vi "Initialize Motor Communication Ref.vi"(8 "error in (no error)":errorcluster, 11 "motor name (unnamed)":string) -> (0 "error out":errorcluster, 3 "motor communication ref out":refnum<class "NI_Robotics_Motor Communication Ref.lvclass">)   [LabVIEW 2017, in "NI_Robotics_Motor Communication Ref.lvclass"]
uses:
  <vilib>/robotics/Actuation/Motor Communication Ref/NI_Robotics_Motor Communication Ref.lvclass
  c:/Program Files (x86)/National Instruments/LabVIEW 2017/vi.lib/robotics/Actuation/Motor Communication/NI_Robotics_Motor Communication.lvclass
  <vilib>/robotics/Actuation/Motor Communication Ref/NI_Robotics_Motor Communication Ref.lvclass/NI_Robotics_Motor Communication Ref.ctl
  <vilib>/robotics/Actuation/Motor Communication/NI_Robotics_Motor Communication.lvclass/NI_Robotics_Motor Communication.ctl
  <vilib>/robotics/Actuation/Motor Communication Ref/FG Motor Comm Ref Sessions Action.ctl
  <vilib>/robotics/Actuation/Motor Communication Ref/Check if Refs are Valid.vi
  <vilib>/robotics/Actuation/Motor Communication/NI_Robotics_Motor Communication.lvclass
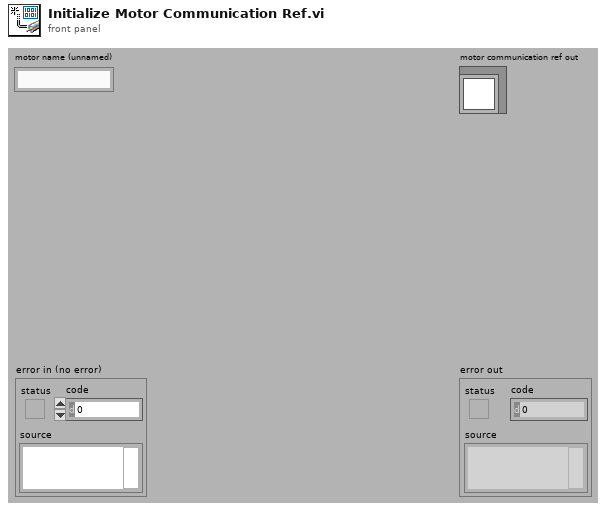
[diagram p1: front panel]
types:
  T1 = typedef "NI_Robotics_Motor Communication Ref.lvclass/FG Motor Comm Ref Sessions Action.ctl" = enum16{"Get", "Add", "Delete"}
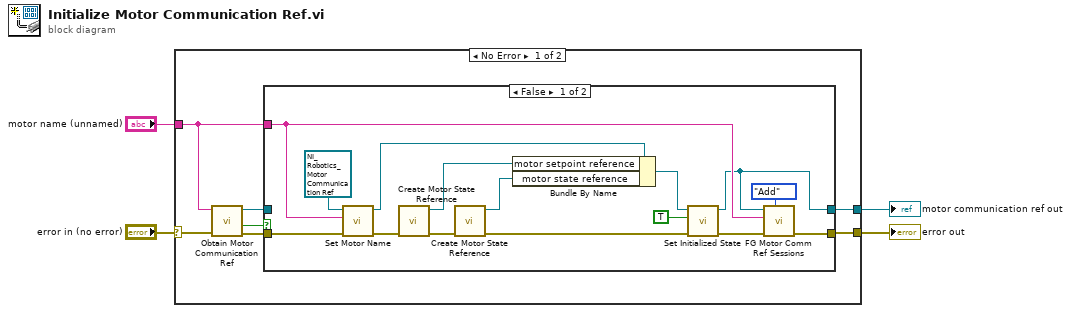
[diagram p0: block diagram]
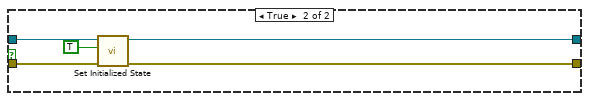
[diagram p2: hidden frame]
diagram:
  n1 = case shown="No Error" "error in (no error)" {
    selector: "error in (no error)" -> [w7 w32]
    tunnel: [w8 w32] -> w3
    tunnel: "motor name (unnamed)" -> [w6 _]
    tunnel: [w5 _] -> w1
    frame No Error {
      n2 = call <vilib>:"Obtain Motor Communication Ref.vi"("error in (no error)"=w7, "motor name"=w6) -> ("error out"=w10:errorcluster, "valid?"=w11:bool, "motor communication ref out"=w9:refnum<class "NI_Robotics_Motor Communication Ref.lvclass">)  [unwired: 7 in]
      n3 = case shown="False" w11 {
        tunnel: w10 -> [w26 w28]
        tunnel: w9 -> [_ w30]
        tunnel: [w19 w27] -> w8
        tunnel: [w15 w29] -> w5
        tunnel: w6 -> [w18 _]
        frame False {
          n4 = call <vilib>:"Set Motor Name.vi"("error in (no error)"=w26, "motor name"=w18, "motor communication in"=refnum<class "NI_Robotics_Motor Communication Ref.lvclass"> refnum ("NI_Robotics_Motor Communication Ref in")) -> ("error out"=w24:errorcluster, "motor communication out"=w22:refnum<class "NI_Robotics_Motor Communication Ref.lvclass">)  [unwired: 7 in]
          n5 = call <vilib>:"Create Motor State Reference.vi"("error in (no error)"=w24) -> ("error out"=w23:errorcluster, "motor state ref"=w20:refnum<data-value>)  [unwired: 9 in]
          n6 = call <vilib>:"Create Motor State Reference.vi"("error in (no error)"=w23) -> ("error out"=w14:errorcluster, "motor state ref"=w21:refnum<data-value>)  [unwired: 9 in]
          n7 = Bundle By Name(cluster=w22, "motor setpoint reference"=w20, "motor state reference"=w21) -> (w16:refnum<class "NI_Robotics_Motor Communication Ref.lvclass">)
          n8 = call <vilib>:"Set Initialized State.vi"("error in (no error)"=w14, "initialized"=TRUE, "motor communication in"=w16) -> ("error out"=w13:errorcluster, "motor communication out"=w15:refnum<class "NI_Robotics_Motor Communication Ref.lvclass">)  [unwired: 7 in]
          n9 = call <vilib>:"FG Motor Comm Ref Sessions.vi"("action"=FG_Motor_Comm_Ref_Sessions_Action."Add", "error in (no error)"=w13, "motor name"=w18, "motor communication ref in"=w15) -> ("error out"=w19:errorcluster)  [unwired: 5 in, 2 out]
        }
        frame True {
          n10 = call <vilib>:"Set Initialized State.vi"("error in (no error)"=w28, "initialized"=TRUE, "motor communication in"=w30) -> ("error out"=w27:errorcluster, "motor communication out"=w29:refnum<class "NI_Robotics_Motor Communication Ref.lvclass">)  [unwired: 7 in]
        }
      }
    }
    frame Error {
    }
  }
  "error out" <- w3
  "motor communication ref out" <- w1
